vi "Increment Count.vi"(8 "error in (no error)":errorcluster, 11 "String Dictionary in":refnum<class "String Database.lvclass">=refnum) -> (0 "error out":errorcluster, 3 "String Dictionary out":refnum<class "String Database.lvclass">)   [LabVIEW 2018, in "String Database.lvlib" / "String Database.lvclass"]
uses:
  String Database.lvclass
  String Database.lvclass/String Database.ctl
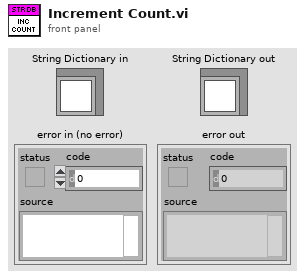
[diagram p1: front panel]
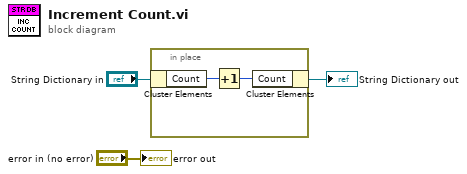
[diagram p0: block diagram]
diagram:
  n1 = in-place {
    n2 = in-place-cluster #1("String Dictionary in") -> ("Count"=w5:i32)
    n3 = Increment(x=w5) -> (x+1=w4:i32)
    n4 = in-place-cluster #1("Count"=w4) -> (→"String Dictionary out":refnum<class "String Database.lvclass">)
  }
  "error out" <- "error in (no error)"
